vi "Actor Core.vi"(8 "error in":errorcluster, 11 "Controller in":refnum<class "Controller.lvclass">) -> (0 "error out":errorcluster, 3 "Actor out":refnum<class "Actor.lvclass">)   [LabVIEW 2019, in "Controller.lvlib" / "Controller.lvclass"]
doc: "(<B>Filename</B>: Actor Framework.lvlib:Actor.lvclass:Actor Core.vi)\n\nReceives messages to the actor, reacts to them, and initiates any error handling that may shut the actor down.\n\nDescendant classes may override this VI to append parallel tasks for the actor to complete while it handles messages. Overrides use the Call Parent Method node."
uses:
  Controller.lvclass
  C:/Program Files (x86)/National Instruments/LabVIEW 2019/vi.lib/ActorFramework/Actor/Actor.lvclass
  <vilib>/ActorFramework/Actor/Actor.lvclass
  Counts.ctl
  Controller Messages/Move Older Unmatched Events Msg/Move Older Unmatched Events Msg.lvclass
  C:/Program Files (x86)/National Instruments/LabVIEW 2019/vi.lib/ActorFramework/Message/Message.lvclass
  <vilib>/ActorFramework/Message Enqueuer/Message Priority.ctl
  Logger/Logger/Logger.lvclass
  <vilib>/ActorFramework/Actor/Actor.lvclass/Actor.ctl
  <vilib>/ActorFramework/Message Enqueuer/Message Enqueuer.lvclass/Message Enqueuer.ctl
  Controller.lvclass/Controller.ctl
  Logger/Logger/Logger.lvclass/Logger.ctl
  Controller Messages/Set Match Window Msg/Set Match Window Msg.lvclass/Set Match Window Msg.ctl
  <vilib>/ActorFramework/Message Enqueuer/Init from Existing Queue.vi
  <vilib>/ActorFramework/Message Enqueuer/Enqueue.vi
  <vilib>/ActorFramework/Stop Msg/Stop Msg.lvclass
  Controller Messages/Set Match Window Msg/Set Match Window Msg.lvclass
  <vilib>/Analysis/1siggen.llb/Ramp Pattern by Delta.vi
  <vilib>/ActorFramework/Message Priority Queue/Priority Enqueue.vi
  <vilib>/ActorFramework/Message Enqueuer/Message Enqueuer.lvclass
  <vilib>/Analysis/NI_AALBase.lvlib
panel:
  out "Slave 'Histogram'":cluster{"X":dbl, "Y":dbl}[](graph)
  out "Master 'Histogram'":cluster{"X":dbl, "Y":dbl}[](graph)
  in  "Time Window (s)":dbl=0.1
  out "Time Expired":dbl
  out "Event Counts":T1 {"Coincident Event Rate" format="%.3g"; "Single Slave Event Rate" format="%.3g"; "Single Master Event Rate" format="%.3g"}
  out "Event ADC Counts Graph":cluster{i32, i32}[](graph)
  # "The histograms show both single and coincident values"
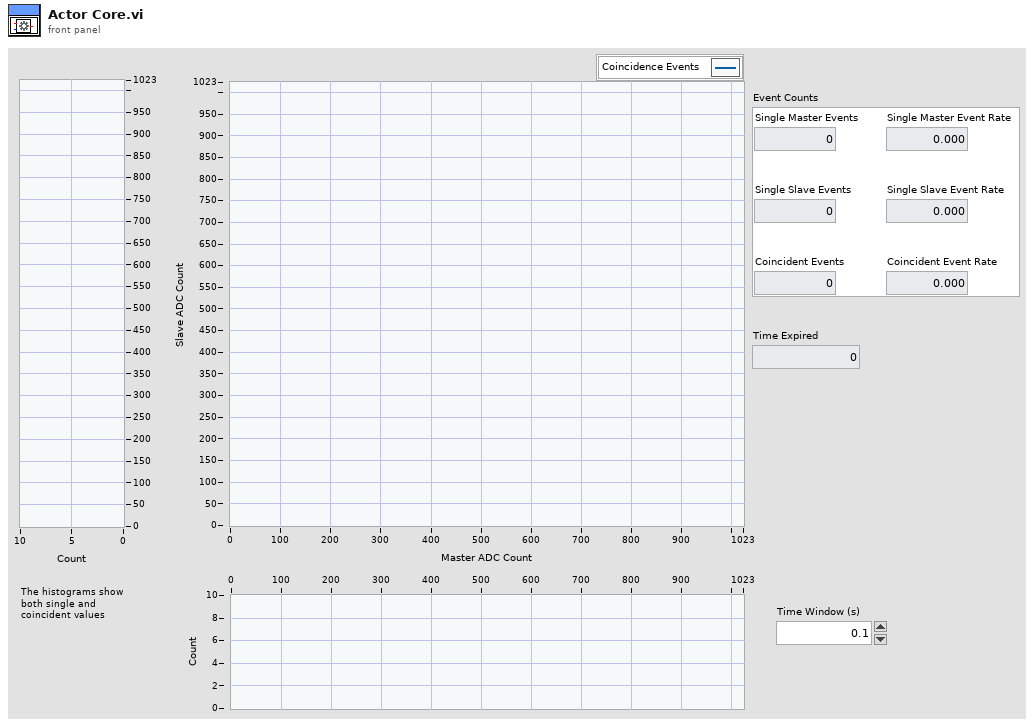
[diagram p1: front panel]
types:
  T1 = typedef "Counts.ctl" = cluster{"Single Master Events":i32, "Single Slave Events":i32, "Coincident Events":i32, "Single Master Event Rate":dbl, "Single Slave Event Rate":dbl, "Coincident Event Rate":dbl}
  T2 = enum32{"Invalid", "Standard", "Closed", "Hidden", "Minimized", "Maximized"}
  T3 = typedef "Actor Framework.lvlib/Message Enqueuer.lvclass/Message Priority.ctl" = enum16{"Low", "Normal", "High"}
  T4 = typedef "imagedata.ctl" = cluster{"image type":i32, "image depth":i32, "image":u8[], "mask":u8[], "colors":u32[], "Rectangle":cluster{"left":i16, "top":i16, "right":i16, "bottom":i16}}
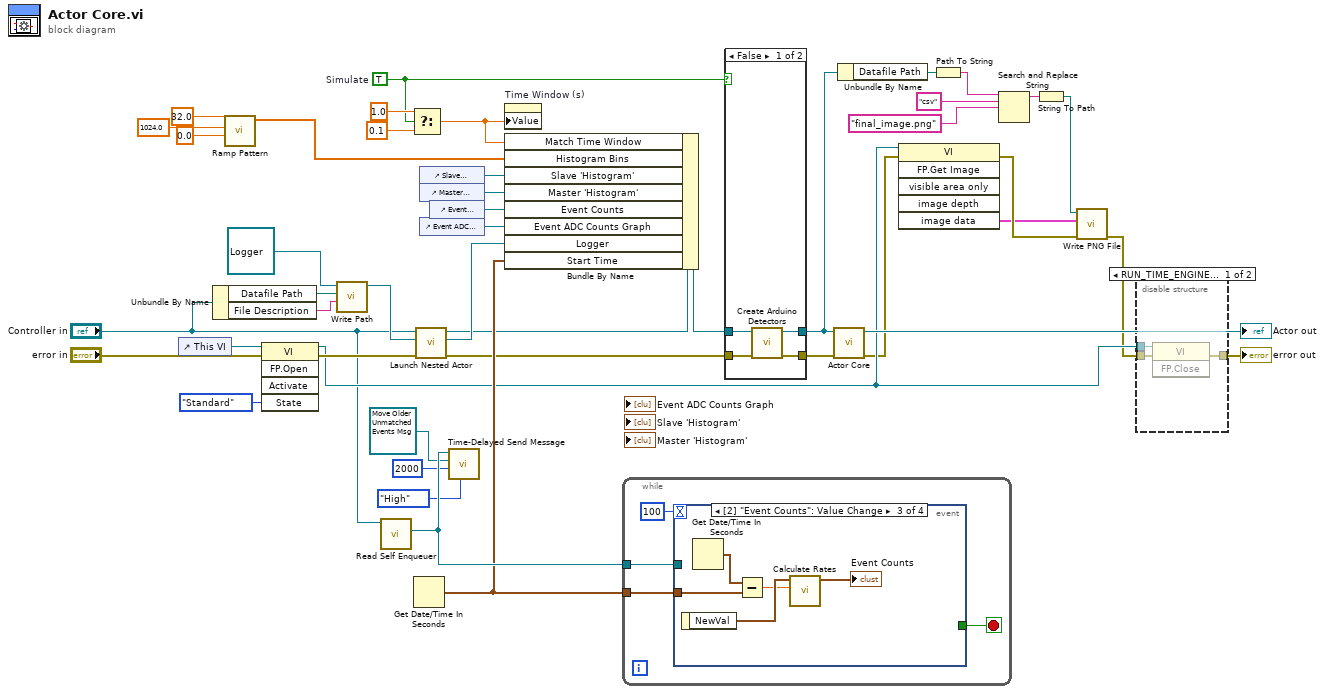
[diagram p0: block diagram]
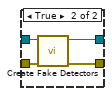
[diagram p3: hidden frame]
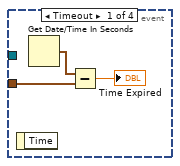
[diagram p4: hidden frame]
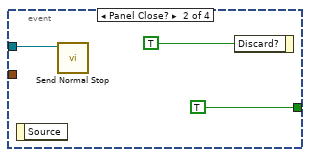
[diagram p5: hidden frame]
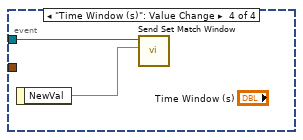
[diagram p6: hidden frame]
diagram:
  w32 = TRUE  # Simulate
  n1 = control-ref of="This VI"() -> (w26:refnum<vi>)
  n2 = Unbundle By Name("Controller in") -> ("Datafile Path"=w2:path, "File Description"=w1:string)
  n3 = call-poly <vilib>:"Ramp Pattern.vi"("start"=0.0, "end"=1024.0, "delta"=32.0) -> ("Ramp Pattern"=w16:dbl[])  [unwired: 6 in, 2 out]
  n4 = invoke class="VI" method="FP.Open"(reference=w26, error in="error in", "State"=T2."Standard") -> (reference out=w14:refnum<vi>, error out=w24:errorcluster)  [unwired: 2 in, 3 out]
  n5 = call "Write Path.vi"("Header Description"=w1, "Path"=w2, "Logger in"=refnum<class "Logger.lvclass"> refnum ("Logger.lvlib:Logger.lvclass")) -> ("Logger out"=w28:refnum<class "Logger.lvclass">)  [unwired: 7 in, 1 out]
  n6 = call <vilib>:"Read Self Enqueuer.vi"("Actor"="Controller in") -> ("Self Enqueuer"=w43:refnum<class "Message Enqueuer.lvclass">)  [unwired: 10 in]
  n7 = Select(t=1.0, s=w32, f=0.1) -> (s? t:f=w20:dbl)
  n8 = Get Date/Time In Seconds() -> (seconds since 1Jan1904=w42:timestamp)
  n9 = call <vilib>:"Launch Nested Actor.vi"("error in (no error)"=w24, "Nested Actor"=w28, "Caller Actor in"="Controller in") -> ("error out"=w31:errorcluster, "Nested Actor's Enqueuer"=w44:refnum<class "Message Enqueuer.lvclass">, "Caller Actor out"=w30:refnum<class "Controller.lvclass">)  [unwired: 6 in]
  n10 = control-ref of="Slave 'Histogram'"() -> (w15:refnum<vi>)
  n11 = control-ref of="Master 'Histogram'"() -> (w21:refnum<vi>)
  n12 = control-ref of="Event ADC Counts Graph"() -> (w40:refnum<vi>)
  n13 = control-ref of="Event Counts"() -> (w27:refnum<vi>)
  n14 = call <vilib>:"Time-Delayed Send Message.vi"("Message Priority (Normal)"=Message_Priority."High", "Milliseconds To Wait"=2000, "Message"=refnum<class "Move Older Unmatched Events Msg.lvclass"> refnum ("Controller.lvlib:Move Older Unmatched Events Msg.lvclass"), "Message Enqueuer"=w43) -> ()  [unwired: 6 in, 2 out]
  n15 = property on="Time Window (s)" class="DigNum (strict)"("Value"=w20) -> ()  [unwired: 2 in, 2 out]
  n16 = Bundle By Name(cluster=w30, "Match Time Window"=w20, "Histogram Bins"=w16, "Slave 'Histogram'"=w15, "Master 'Histogram'"=w21, "Event Counts"=w27, "Event ADC Counts Graph"=w40, "Logger"=w44, "Start Time"=w42) -> (w36:refnum<class "Controller.lvclass">)
  n17 = while {
    tunnel: w42 -> [w48]
    tunnel: w43 -> [w46]
    stop <- w47 stop-if-true
    n18 = event shown="[2] \"Event Counts\": Value Change" {
      selector: _ -> [_ _ _ _]
      dyn-events: _ -> [_ _ _ _]
      timeout: 100 -> [_ _ _ _]
      tunnel: w48 -> [w51 _ w59 _]
      tunnel: [_ TRUE _ _] -> w47
      tunnel: w46 -> [_ w53 _ w62]
      event Timeout {
        n19 = event-data() -> ()  [unwired: 1 in, 1 out]
        n20 = Get Date/Time In Seconds() -> (seconds since 1Jan1904=w52:timestamp)
        n21 = Subtract(x=w52, y=w51) -> (x-y=→"Time Expired":dbl)
      }
      event Panel Close? {
        n22 = event-data() -> ()  [unwired: 1 in, 1 out]
        n23 = call <vilib>:"Send Normal Stop.vi"("Message Enqueuer"=w53) -> ()  [unwired: 10 in, 1 out]
        n24 = event-data("Discard?"=TRUE) -> ()  [unwired: 1 in, 1 out]
      }
      event Value Change {
        n25 = event-data() -> ("NewVal"=w58:T1)  [unwired: 1 in]
        n26 = Get Date/Time In Seconds() -> (seconds since 1Jan1904=w60:timestamp)
        n27 = Subtract(x=w60, y=w59) -> (x-y=w57:dbl)
        n28 = call "Calculate Rates.vi"("Duration (s)"=w57, "Event Counts"=w58) -> ("Event Counts with Rate"=→"Event Counts":T1)  [unwired: 9 in]
      }
      event "Time Window (s)": Value Change {
        n29 = event-data() -> ("NewVal"=w61:dbl)  [unwired: 1 in]
        n30 = call "Send Set Match Window.vi"("Match Time Window"=w61, "Message Enqueuer"=w62) -> ()  [unwired: 8 in, 2 out]
      }
    }
  }
  n31 = case shown="False" w32 {
    tunnel: w36 -> [w66 w70]
    tunnel: w31 -> [w65 w69]
    tunnel: [w64 w68] -> w12
    tunnel: [w63 w67] -> w35
    frame False {
      n32 = call "Create Arduino Detectors.vi"("error in (no error)"=w65, "Controller in"=w66) -> ("error out"=w63:errorcluster, "Controller out"=w64:refnum<class "Controller.lvclass">)  [unwired: 8 in]
    }
    frame True {
      n33 = call "Create Fake Detectors.vi"("error in (no error)"=w69, "Controller in"=w70) -> ("error out"=w67:errorcluster, "Controller out"=w68:refnum<class "Controller.lvclass">)  [unwired: 8 in]
    }
  }
  n34 = call-parent "Actor Core.vi"("error in"=w35, "Actor in"=w12) -> ("error out"=w5:errorcluster, "Actor out"=→"Actor out":refnum<class "Actor.lvclass">)  [unwired: 8 in]
  n35 = Unbundle By Name(w12) -> ("Datafile Path"=w11:path)
  n36 = invoke class="VI" method="FP.Get Image"(reference=w14, error in=w5) -> (error out=w45:errorcluster, "image data"=w13:T4)  [unwired: 4 in, 4 out]
  n37 = Path To String(path=w11) -> (string=w10:string)
  n38 = Search and Replace String(input string=w10, search string="csv", replace string="final_image.png" ("replace string (\"\")")) -> (result string=w9:string)  [unwired: 5 in, 3 out]
  n39 = String To Path(string=w9) -> (path=w8:path)
  n40 = call <vilib>:"Write PNG File.vi"("error in (no error)"=w45, "image data"=w13, "path to PNG file"=w8) -> ("error out"=w4:errorcluster)  [unwired: 7 in, 1 out]
  n41 = disable-structure shown="RUN_TIME_ENGINE==True" {
    disable-tunnel: w4 -> [w73 w74]
    disable-tunnel: [w72 w74] -> w22
    disable-tunnel: w14 -> [w71 _]
    frame condition #0 {
      n42 = invoke class="VI" method="FP.Close"(reference=w71, error in=w73) -> (error out=w72:errorcluster)  [unwired: 1 in, 2 out]
    }
    frame condition #1 (active) {
    }
  }
  "error out" <- w22
